vi "Process each line scan-STFT.vi"() -> ()   [LabVIEW 2012]
uses:
  <vilib>/Analysis/3filter.llb/Filter Passband Type.ctl
  <vilib>/addons/Time Frequency Analysis/Spectrogram.llb/TFA STFT Spectrogram (Real).vi
  <vilib>/addons/_Advanced Signal Processing/NI_AdvSigProcTFA.lvlib
  <vilib>/Analysis/NI_AALBase.lvlib
panel:
  in  "y":dbl
  out "Sampling":dbl=20.108695652173914
  out "Normal data 2":dbl[](graph)=[0.0834075791833563, 0.08313970177121038, 0.0834899535484272, 0.08389902003780546, 0.08427136598221668, 0.08461348581592272, 0.08492340251028675, 0.08521667523546025, 0.0851111968881446, 0.08489623450777979, 0.08467501600489258, 0.08449341136165812, 0.08438920507645266, 0.08460003202327245, 0.08510447184853119, 0.08579713933260916, 0.08653197427791655, 0.08705551964151328, 0.08731618076837931, 0.08700373675029589, 0.08672696237995277, 0.08664592369200513, 0.08655582285594121, 0.08621897822172135, 0.08561574308478548, 0.08491342099016591, 0.08460246301489456, 0.08478803233150298, 0.0854502734325155, 0.08654879942246066, 0.08755712035158278, 0.08840500364883493, 0.08889951751029518, 0.08912122981771826, 0.08918683174411485, 0.08898115715259142, 0.08876739958002902, 0.08855711942154582, 0.08823290404160386, 0.08796266023610444, 0.08780370630349933, 0.08782190555450581, 0.08779942707995848, 0.08765856529004035, 0.0877601550773121, 0.08799573666984463, 0.08826219785854382, 0.08847733504567026, 0.08827829100091344, 0.08803405876562488, 0.08781825439049842, 0.08755912193194208, 0.08713062620335557, 0.08672690059093638, 0.08637632341089246, 0.08635609835576827, 0.0866510131576495, 0.0871786545522629, 0.08791692308970493, 0.0885621644918122, 0.08879620456503601, 0.08872932271408505, 0.08850747747035358, 0.0882542830304037, 0.08787707433351256, 0.08761851428242066, 0.08748244344771558, 0.0875997776510181, 0.0877097458591143, 0.08794689348266707, 0.08821061524956454, 0.08849169338933487, 0.08886172810529823, 0.08915641172303683, 0.0893067619524749, 0.08922040922761751, 0.0888805318841088, 0.08828348331667667, 0.08788362391897823, 0.08793840721039217, 0.08824789785389507, 0.08862514612141138, 0.08883206039491341, 0.08898326194563837, 0.08913917759091769, 0.08916247582719061, 0.08903372800703718, 0.08907598505484265, 0.08923405396793974, 0.08964928973562009, 0.08985769352605168, 0.0899889448460994, 0.08997252723056448, 0.09003444243961788, 0.09000387785810496, 0.08974740294044986, 0.08951832066608535, 0.08930260883466949, 0.08921838638817513, 0.08934557688893602, 0.08946284735612371, 0.08960602453208318, 0.08960524390657572, 0.08958575680786628, 0.08939154000736746, 0.08914838070882043, 0.08893965118076647, 0.08877081744441315, 0.08871181747889478, 0.08874766542518792, 0.08894066907473949, 0.0890407674789974, 0.08917440557162377, 0.08929194722397699, 0.0894254391850194, 0.08965318224027374, 0.08975994361406868, 0.08983908154185455, 0.08975676345341065, 0.0896655189776547, 0.08962187443800529, 0.0894548374413544, 0.0894140129850669, 0.08934585208487401, 0.08931804020086846, 0.08931011814499568, 0.08935279460412285, 0.08945028571146957, 0.08957184114621686, 0.08969807375334708, 0.08988845373764943, 0.0899716889936294, 0.090089696720983, 0.09021449147086749, 0.09020310093423652, 0.08991848453175759, 0.0894937239984702, 0.08917733895602646, 0.08899709326825977, 0.08892540375977825, 0.0890035549544317, 0.08908530759728554, 0.0892475643640946, 0.08939033012753242, 0.08927946471364707, 0.08935697041978198, 0.08934658967569127, 0.08931773331801529, 0.08913863456394741, 0.08883605628176924, 0.08858816340341268, 0.08853329089933158, 0.08867196316811013, 0.08896796964724031, 0.08952338206501471, 0.09009322119402816, 0.0905595365183964, 0.09080113581397806, 0.0909438406240406, 0.09089973654160234, 0.09075310482709704, 0.09061553000362736, 0.09065965018843884, 0.09075070943262445, 0.0908072787852049, 0.0908406571589153, 0.09087777000386214, 0.09091673158353443, 0.09099736410774313, 0.09098086369104644, 0.09095028163485372, 0.09092432740621845, 0.09085355749675111, 0.090863062942775, 0.09078508334197923, 0.09078572200755262, 0.09076354138299104, 0.09068778307670722, 0.0906211966896475, 0.09063357076790778, 0.0905736920984023, 0.09062786145822013, 0.09064631440011012, 0.09075874804311274, 0.09090496519552399, 0.09096196397969845, 0.09098103219650104, 0.09101335257201719, 0.09105649854110265, 0.0911834152497393, 0.09161578233100716, 0.09217231896964619, 0.09222971534791932, 0.09225759430868143, 0.09209598933915224, 0.09168598727057885, 0.09099377580514717, 0.090186042411056, 0.0894481411133792, 0.08915981262879302, 0.08912425301719222, 0.08944704248945372, 0.08989058542377173, 0.09033264071795759, 0.09078708163321099, 0.091098895952144, 0.09121182762732068, 0.09126419254960312, 0.09115060183968558, 0.09106063737983011, 0.09084827667605727, 0.09066749446496715, 0.09042351312787533, 0.09040410584458498, 0.09045351002567686, 0.09056800939596742, 0.09076101702089538, 0.09131981273651768, 0.09168050695075432, 0.09162024786173475, 0.09161211882919608, 0.09130426204675211, 0.09111404350435864, 0.09091646587709575, 0.0907416229021263, 0.09059513303092509, 0.09059034346057933, 0.09062428441173002, 0.09068272665571606, 0.09076796159454331, 0.09095305396878844, 0.09097950357072662, 0.0910677086901931, 0.09099903293507541, 0.09101945384291224, 0.09095861492796396, 0.09075473312906945, 0.0905358760350409, 0.09027851944412824, 0.09026508064463204, 0.09052018817428631, 0.09085182601186455, 0.09113570967206829, 0.09140447267373093, 0.09138131324528526, 0.09128743494948562, 0.09113422354215352, 0.09087067415893002, 0.0904679203104334, 0.08982267543983533, 0.08928259181492867, 0.08905952402546756, 0.0889948658461748, 0.08914842305527344, 0.08937270201093563, 0.08977928982849018, 0.09014773107526487, 0.09038887112593925, 0.09066164060514795, 0.09092713557691277, 0.09115380669134177, 0.09125394414334624, 0.09125093559392046, 0.09120699051484178, 0.09113870117656733, 0.09112001814240331, 0.09122754606725744, 0.09158688873184688, 0.09165592260252194, 0.09178788763588348, 0.09180930100747726, 0.09190329878534668, 0.092084321043552, 0.09213522227247237, 0.09216730307160437, 0.09215936139295011, 0.09208864889102408, 0.09201867372083274, 0.09195030260091844, 0.09173073709383099, 0.09128048297964311, 0.09093544261044752, 0.09073962740515583, 0.09087511467887456, 0.09123225293936388, 0.09150648815959149, 0.09156727601686483, 0.09147265783843454, 0.0914111402191003, 0.0911916715797567, 0.0909712570516758, 0.09072504742815508, 0.09061970963347508, 0.09063096143272416, 0.0907745502789912, 0.09107791843520448, 0.09131583724609288, 0.09133734081948365, 0.09116819781953764, 0.09109715216909342, 0.0910423293862588, 0.09087411894711536, 0.09063123724373874, 0.09039356922638893, 0.09016409878067437, 0.08997533063897944, 0.08994298805661663, 0.08989425302147865, 0.0899207350403956, 0.08992246364934127, 0.09013591069051792, 0.09033620829615385, 0.09048717601286119, 0.0906934564023864, 0.09104347398847805, 0.09147302683649448, 0.09179476309009273, 0.09181671888542828, 0.09163891829611832, 0.0913741439295705, 0.09111343050349047, 0.09113811314714358, 0.09116985095592305, 0.09095693798237577, 0.090239145728342, 0.0898552913724986, 0.0894963513225219, 0.08922680674023609, 0.08925878186943818, 0.08937129029963889, 0.08938451862761111, 0.08939912934087578, 0.089485920077269, 0.0898145871700708, 0.09027093166136683, 0.0909295746939482, 0.09154241113556146, 0.09180137266982405, 0.0915045644434099, 0.09094416558840128, 0.09038467347996912, 0.09006811267456377, 0.09007771774793784, 0.09037059900020229, 0.09094282972798715, 0.09144898539316408, 0.09179754065889242, 0.09193296778150714, 0.09207085516898232, 0.09211386881896015, 0.09205979362090227, 0.09185704935602204, 0.09160839197725171, 0.09143448063032047, 0.09129095338526669, 0.09123287905762438, 0.09126833752197877, 0.09135545456888215, 0.09163107320936356, 0.09188662501710237, 0.09211903469537222, 0.09238655483907245, 0.09257874234948117, 0.09304342601803188, 0.09331933532641673, 0.09345715850395474, 0.09309942148966914, 0.0926613441226984, 0.09211482272105052, 0.09159102545470406, 0.09107760996181134, 0.09082853222296186, 0.09082629569803746, 0.09075237871250016, 0.09076265776447252, 0.09098839226004328, 0.09128166412524844, 0.09177847463368746, 0.09217072818710526, 0.09217517693702303, 0.09191808105841939, 0.09158255017233621, 0.09129975199003484, 0.0911362664117092, 0.0910101459234221, 0.09086667037505883, 0.09073411102222709, 0.0906738484031689, 0.09078338967697815, 0.09093118267179665, 0.09111917693117444, 0.09122762363626072, 0.09120970954838045, 0.09118435581097911, 0.09100500678245758, 0.09085558830322499, 0.09086395856266347, 0.09075230062315899, 0.09087346503607335, 0.09087066459426082, 0.0908338769279338, 0.09061697191621793, 0.0905142650895385, 0.09004436607888379, 0.08984645925183149, 0.08982998647295336, 0.08972220915887183, 0.08958119771738406, 0.0895114428193082, 0.08956031308318181, 0.08972294987436441, 0.0898267921022315, 0.08986223085653477, 0.0898753763122414, 0.08978378527156854, 0.08967739441348804, 0.0898514788991922, 0.08981954985646216, 0.08966741171024556, 0.0893058551872219, 0.08907296376511623, 0.08909827056134634, 0.08922882767265133, 0.0895372690347607, 0.0899677019420076, 0.09044291501892017, 0.09072700758013175, 0.09078120367841964, 0.0909525232882357, 0.09119892458758112, 0.09152441088405014, 0.0916669657119925, 0.09117299188478313, 0.0909959094356686, 0.09082949582542518, 0.09019081652259521, 0.08947979477594711, 0.08877364402760415, 0.08842704421178378, 0.08833830204511177, 0.08839788284754788, 0.08841244312962042, 0.08853678558187465, 0.08889234989031575, 0.08957362133613204, 0.09021979362675236, 0.09062753774477246, 0.09076979076414887, 0.09073442693129163, 0.09056215420055153, 0.09046273573836079, 0.09055982041513243, 0.09052120452561604, 0.09049447683264696, 0.09043490885526731, 0.09037243190972516, 0.09039319399560133, 0.09038124565272496, 0.09045343383456332, 0.09053446410592082, 0.09068739782157302, 0.09090459329876409, 0.09104500692517432, 0.09120192010204776, 0.09093369673574528, 0.09078223402442004, 0.09074519826617564, 0.09064654637840659, 0.09062798512438529, 0.09061047338978868, 0.09068266583513598, 0.09071418397171756, 0.0907277790026475, 0.0907518201317747, 0.09062977076574907, 0.09078664141797464, 0.09092883726786183, 0.09095381296563722, 0.09093066310699459, 0.09073319935672125, 0.09054126871986297, 0.09054466415507471, 0.09063790643680167, 0.0908011863593963, 0.09072702264485157, 0.09060894238587354, 0.0905200571191692, 0.09052718886347938, 0.09068150334566266, 0.09061283113100234, 0.09045830601418663, 0.09018300568877634, 0.09008439303842755, 0.09015569269002399, 0.09027912731265884, 0.09024778755308062, 0.09020789092533668, 0.09018782971323624, 0.09015446124198573, 0.09010464066539416, 0.08995559964073951, 0.08974841562513391, 0.08952321185010585, 0.08937674069340501, 0.08918782897939286, 0.08906989345691, 0.08894164948590912, 0.08891800331781897, 0.08891665149385067, 0.0890160805487759, 0.0890830771962533, 0.08913137376733951, 0.0890220557498708, 0.088913674618483, 0.08879083068327101, 0.08867519279113113, 0.08861369284994827, 0.08849900873106765, 0.0885032571547728, 0.08858334753272176, 0.08857553029832102, 0.08840924991335808, 0.08823519823807159, 0.0881207970252026, 0.0880141880835164, 0.08799160519748125, 0.08784999274390047, 0.08771920867882962, 0.0875795567180764, 0.08734069452795593, 0.0871103303218063, 0.08656679412466856, 0.08600040359551805, 0.08577927895883158, 0.08612392959476711, 0.08685488657644315, 0.0874467209881569, 0.08762324924646843, 0.08743618643489552, 0.08714840902575245, 0.08683686333626603, 0.08670386834306683, 0.08659863168439075, 0.08635880087590013, 0.08617229184961968, 0.085988483905674, 0.08573275310653554, 0.08538148598015705, 0.08487708758946282, 0.0844201123816035, 0.08422523268656287, 0.08417934269529112, 0.08411207259082858, 0.08401874979189045, 0.08404000557719687, 0.08408975494168326, 0.08421892639457558, 0.08418894696807569, 0.0841036190406738, 0.08391463750273015, 0.08377866932582091, 0.0836375839374231, 0.08359934478547806, 0.08357095823570675, 0.08361020928420444, 0.08365173621804899, 0.08361463365424275, 0.08351551486747148, 0.08334456736979802, 0.08314259168235283, 0.08302723373749957, 0.08308501755828071, 0.08321198578495582, 0.08343324221931987, 0.0838572065524355, 0.08425262508526975, 0.08422266832129416, 0.08425959187247681, 0.08376815407906621]
  in  "Scan length(mm)":dbl=230.0
  in  "window info":cluster{"type":i32, "length":i32}={"type"=1, "length"=8} {"type" items=["None ", "Hanning", "Hamming", "Blackman-Harris", "Exact Blackman", "Blackman", "Flat Top", "4 Term B-Harris ", "7 Term B-Harris", "Low Sidelobe", "Gaussian"]}
  in  "time-frequency sampling info":cluster{"time steps":i32, "frequency bins":i32}={"time steps"=8, "frequency bins"=512}
  in  "CH":i32
  out "STFT Spectrogram":dbl[][](graph)
  in  "filter type":T1
  in  "High Cutoff Freq":dbl=300.0
  in  "Offset Diff":dbl=2.0
  in  "Offset Normal":dbl=2.0
  out "Differential data":dbl[][](graph)
  out "Normal data":dbl[][](graph)
  in  "Low Cutoff Freq":dbl=50.0
  in  "Open":bool
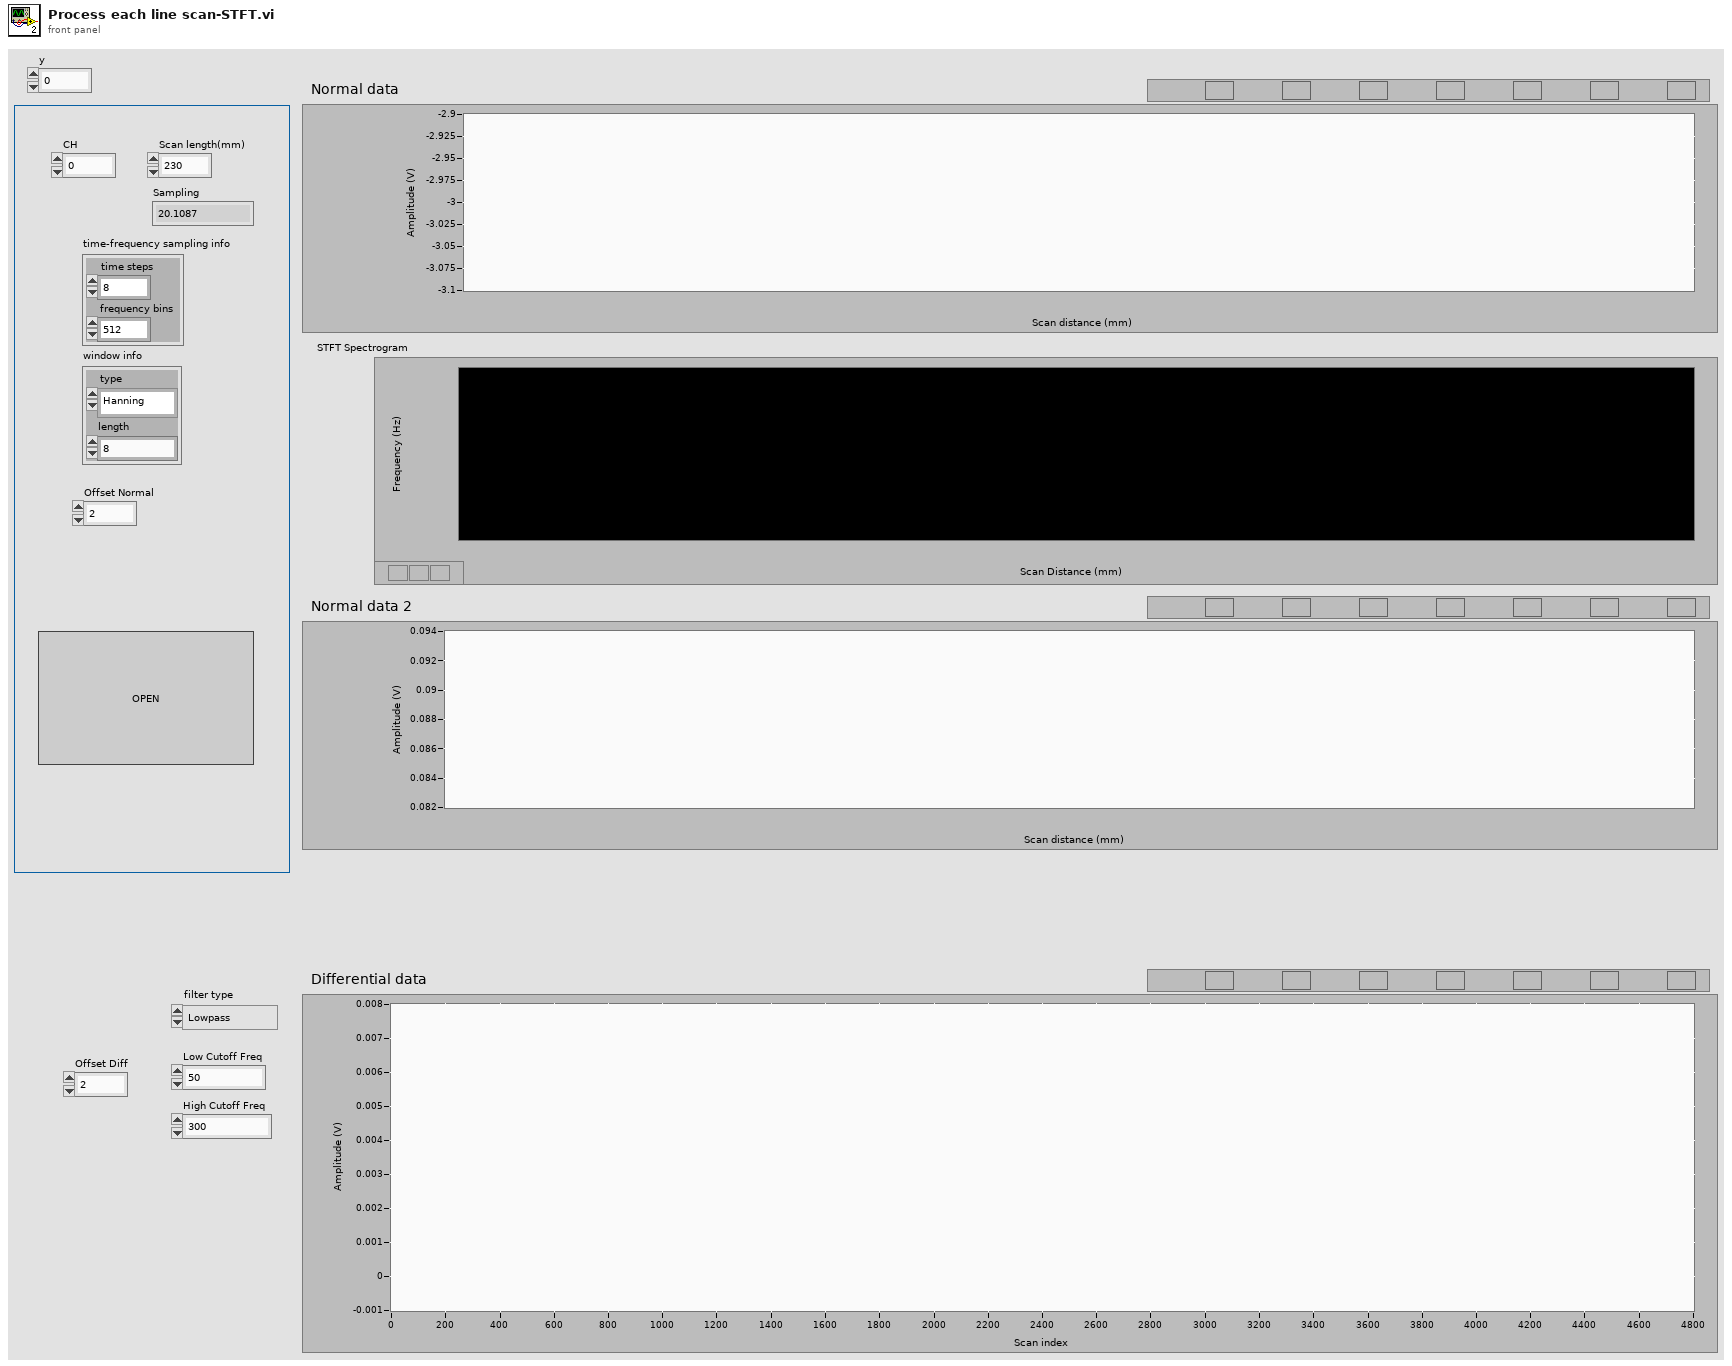
[diagram p1: front panel]
types:
  T1 = typedef "NI_AALBase.lvlib/Filter Passband Type.ctl" = enum32{"Lowpass", "Highpass", "Bandpass", "Bandstop"}
  T2 = cluster{"frequency offset":dbl, "frequency multiplier":dbl}
  T3 = cluster{"time offset":dbl, "time multiplier":dbl}
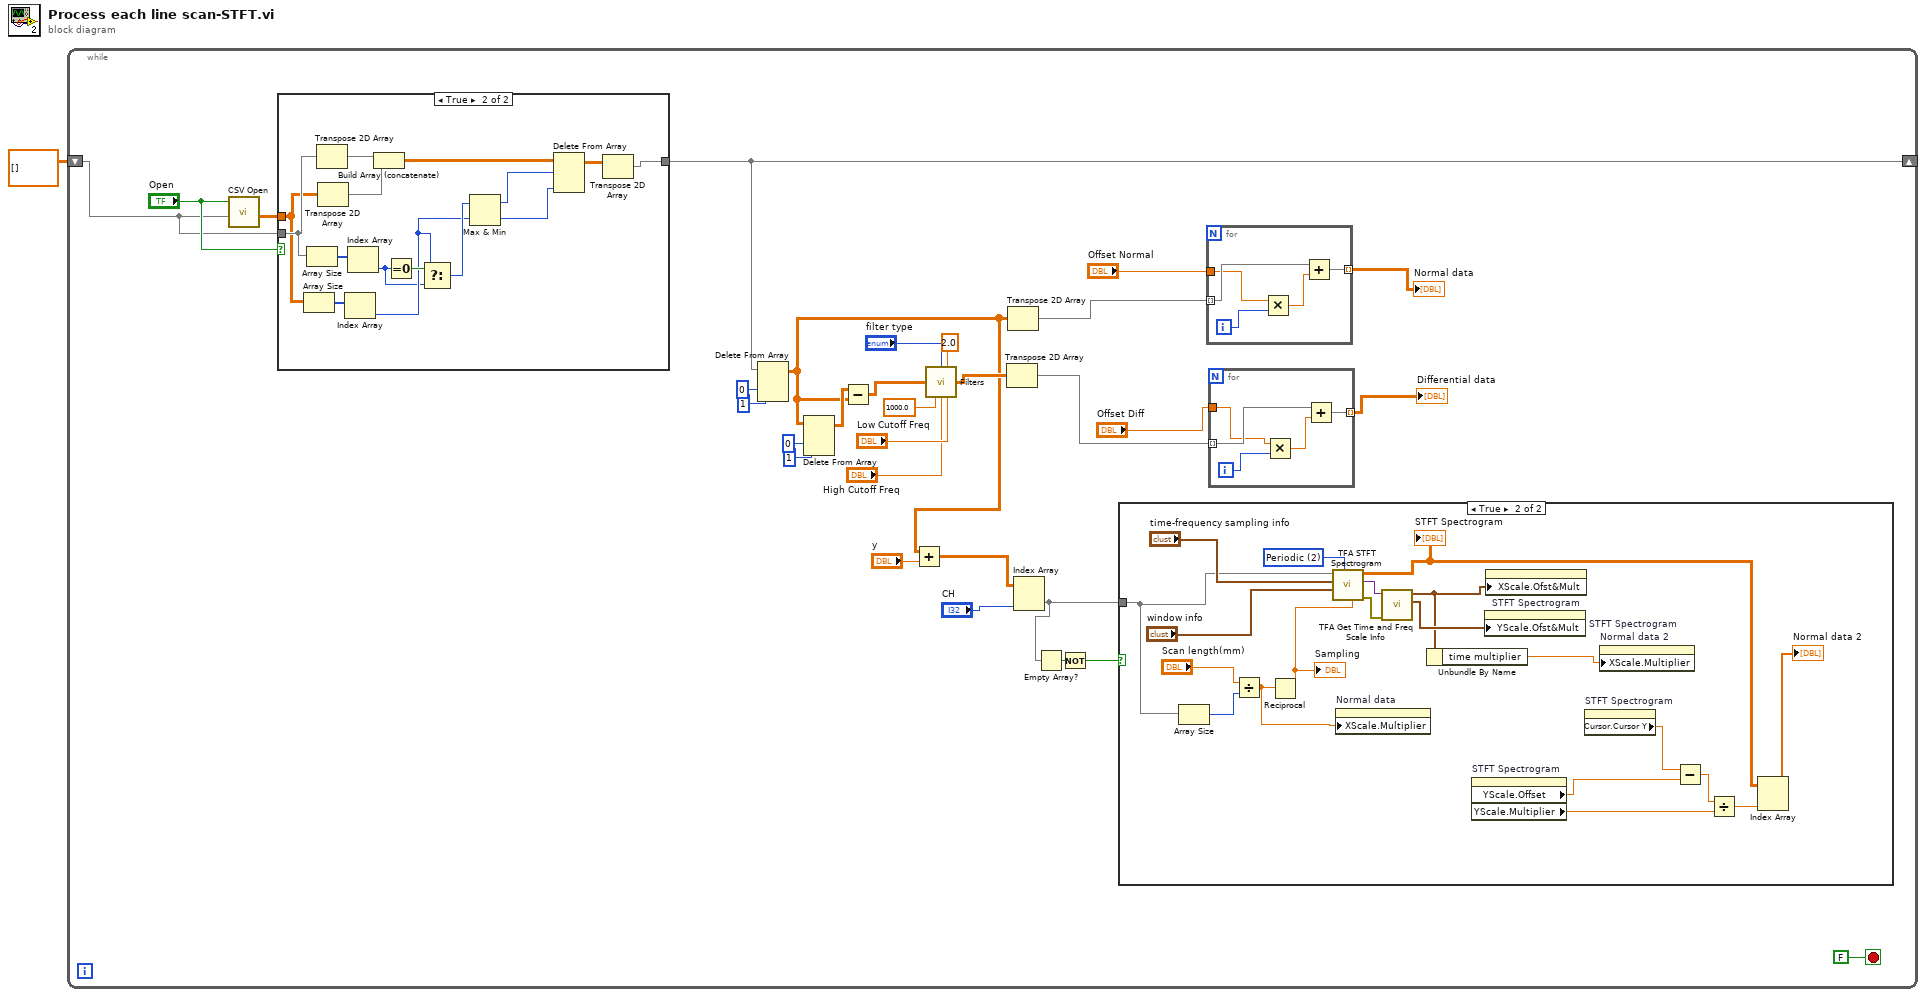
[diagram p0: block diagram]
diagram:
  n1 = while {
    shift-right: [w18] -> _
    shift-left: dbl[][] [] ("2D Array Out") -> [w19]
    stop <- FALSE stop-if-true
    n2 = call "CSV Open.vi"("2D Array In"=w19, "Open"="Open") -> ("2D Array Out"=w20:dbl[][])  [unwired: 9 in]
    n3 = case shown="True" "Open" {
      tunnel: [w62 w69] -> w18
      tunnel: w20 -> [w62 w72]
      tunnel: w19 -> [_ w75]
      frame False {
      }
      frame True {
        n4 = Array Size(array=w72) -> (size(s)=w73:i32[])
        n5 = Array Size(array=w75) -> (size(s)=w74:i32[])
        n6 = Transpose 2D Array(2D array=w75) -> (transposed array=w77:dbl[][])
        n7 = Transpose 2D Array(2D array=w72) -> (transposed array=w76:dbl[][])
        n8 = Index Array(array=w73) -> (element=w64:i32)  [unwired: 1 in]
        n9 = Index Array(array=w74) -> (element=w63:i32)  [unwired: 1 in]
        n10 = Build Array (concatenate)(w77, w76) -> (w71:dbl[][])
        n11 = Equal To 0?(x=w63) -> (x = 0?=w66:bool)
        n12 = Select(t=w64, s=w66, f=w63) -> (s? t:f=w65:i32)
        n13 = Max & Min(x=w65, y=w64) -> (max(x,y)=w68:i32, min(x,y)=w67:i32)
        n14 = Delete From Array(array=w71, length=w68, index (col)=w67) -> (array with subset deleted=w70:dbl[][])  [unwired: 1 in, 1 out]
        n15 = Transpose 2D Array(2D array=w70) -> (transposed array=w69:dbl[][])
      }
    }
    n16 = Delete From Array(array=w18, length=1 ("길이"), index (row)=0 ("인덱스 (행)")) -> (array with subset deleted=w3:dbl[][])  [unwired: 1 in, 1 out]
    n17 = Delete From Array(array=w3, length=1 ("길이"), index (row)=0 ("인덱스 (행)")) -> (array with subset deleted=w26:dbl[][])  [unwired: 1 in, 1 out]
    n18 = Subtract ("Subtract.vi")(x=w26, y=w3) -> (x-y=w30:dbl[][])
    n19 = Add(x=w3, y="y") -> (x+y=w2:dbl[][])
    n20 = call "Filters.vi"("filter type"="filter type", "Order"=2.0, "Array in"=w30, "Sampling Freq"=1000.0, "High Cutoff Freq"="High Cutoff Freq", "Low Cutoff Freq"="Low Cutoff Freq") -> ("Array out"=w31:dbl[][])  [unwired: 9 in]
    n21 = Transpose 2D Array(2D array=w31) -> (transposed array=w12:dbl[][])
    n22 = Transpose 2D Array(2D array=w3) -> (transposed array=w15:dbl[][])
    n23 = Index Array(array=w2, index (col)="CH") -> (element=w7:dbl[])  [unwired: 1 in]
    n24 = Empty Array?(array=w7) -> (empty?=w6:bool)
    n25 = Not(x=w6) -> (.not. x?=w5:bool)
    n26 = case shown="True" w5 {
      tunnel: w7 -> [_ w49]
      frame False {
      }
      frame True {
        w39 = u16 2 items=["Zero padding", "Symmetric", "Periodic"] ("extension")
        n27 = Array Size(array=w49) -> (size(s)=w46:i32)
        n28 = Divide(x="Scan length(mm)", y=w46) -> (x/y=w40:dbl)
        n29 = Reciprocal(x=w40) -> (1/x=w41:dbl)
        "Sampling" <- w41
        n30 = call-poly <vilib>:"TFA STFT Spectrogram.vi"("sampling rate"=w41, "extension"=w39, "window info"="window info", "time-frequency sampling info"="time-frequency sampling info", "signal"=w49) -> ("error out"=w48:errorcluster, "scale info"=w47:variant, "spectrogram"=w38:dbl[][])  [unwired: 4 in]
        "STFT Spectrogram" <- w38
        n31 = property on="Normal data" class="WFGraph (strict)"("XScale.Multiplier"=w40) -> ()  [unwired: 2 in, 2 out]
        n32 = call <vilib>:"TFA Get Time and Freq Scale Info.vi"("error in (no error)"=w48, "scale info"=w47) -> ("frequency info"=w34:T2, "time info"=w33:T3)  [unwired: 7 in, 1 out]
        n33 = Unbundle By Name(w33) -> ("time multiplier"=w32:dbl)
        n34 = property on="STFT Spectrogram" class="IntGraph (strict)"() -> ("YScale.Offset"=w44:dbl, "YScale.Multiplier"=w43:dbl)  [unwired: 2 in, 2 out]
        n35 = property on="STFT Spectrogram" class="IntGraph (strict)"("YScale.Ofst&Mult"=w34) -> ()  [unwired: 2 in, 2 out]
        n36 = property on="STFT Spectrogram" class="IntGraph (strict)"("XScale.Ofst&Mult"=w33) -> ()  [unwired: 2 in, 2 out]
        n37 = property on="STFT Spectrogram" class="IntGraph (strict)"() -> ("Cursor.Cursor Y"=w37:dbl)  [unwired: 2 in, 2 out]
        n38 = property on="Normal data 2" class="WFGraph (strict)"("XScale.Multiplier"=w32) -> ()  [unwired: 2 in, 2 out]
        n39 = Subtract(x=w37, y=w44) -> (x-y=w42:dbl)
        n40 = Divide(x=w42, y=w43) -> (x/y=w35:dbl)
        n41 = Index Array(array=w38, index (col)=w35) -> (element=→"Normal data 2":dbl[])  [unwired: 1 in]
      }
    }
    n42 = for {
      tunnel: "Offset Normal" -> [w57]
      tunnel: w15 -> [w58] mode=indexing
      tunnel: [w59] -> w14 mode=indexing
      i -> [w61]
      n43 = Multiply(x=w57, y=w61) -> (x*y=w60:dbl)
      n44 = Add(x=w58, y=w60) -> (x+y=w59:dbl[])
    }
    "Normal data" <- w14
    n45 = for {
      tunnel: "Offset Diff" -> [w52]
      tunnel: w12 -> [w53] mode=indexing
      tunnel: [w54] -> w11 mode=indexing
      i -> [w56]
      n46 = Multiply(x=w52, y=w56) -> (x*y=w55:dbl)
      n47 = Add(x=w53, y=w55) -> (x+y=w54:dbl[])
    }
    "Differential data" <- w11
  }
